vi "List-Swap Select and Un-Select.vi"(8 "error in (no error)":errorcluster, 11 "List in":refnum<vi>) -> (0 "error out":errorcluster, 3 "List Out":refnum<vi>)   [LabVIEW 2024]
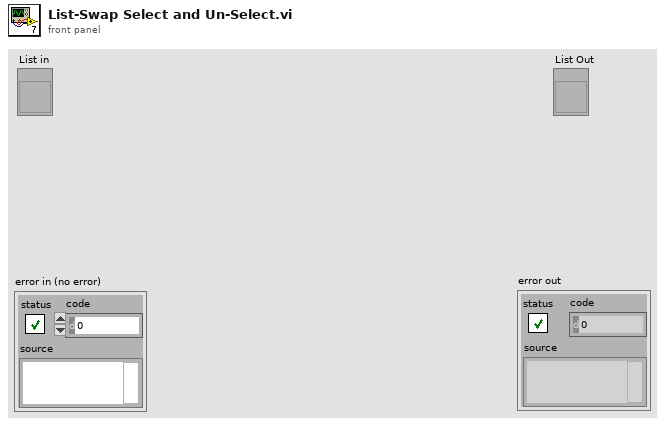
[diagram p1: front panel]
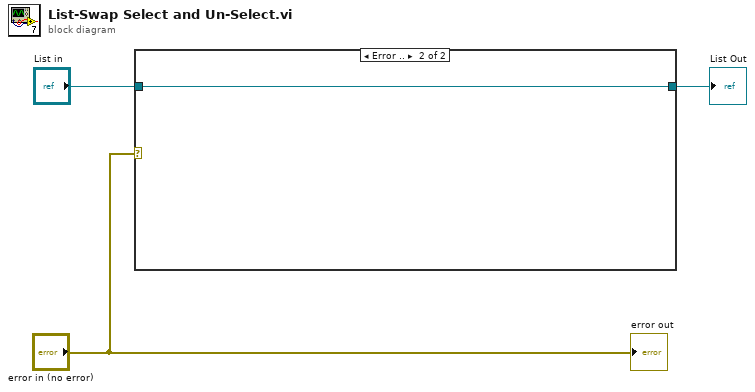
[diagram p0: block diagram]
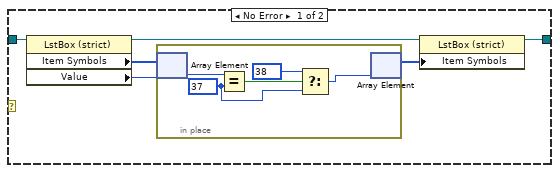
[diagram p2: hidden frame]
diagram:
  n1 = case shown="Error .." "error in (no error)" {
    tunnel: "List in" -> [w5 w15]
    tunnel: [w4 w15] -> w2
    frame No Error {
      n2 = property class="LstBox (strict)"(reference=w5) -> (reference out=w7:refnum<vi>, "Item Symbols"=w9:i32[], "Value"=w8:i32)  [unwired: 1 in, 1 out]
      n3 = in-place {
        w12 = 37
        n4 = in-place-array #1(w9, w8) -> (w14:i32)
        n5 = Equal?(x=w14, y=w12) -> (x = y?=w13:bool)
        n6 = Select(t=38, s=w13, f=w12) -> (s? t:f=w10:i32)
        n7 = in-place-array #1(w10) -> (w6:i32[])  [unwired: 1 out]
      }
      n8 = property class="LstBox (strict)"(reference=w7, "Item Symbols"=w6) -> (reference out=w4:refnum<vi>)  [unwired: 1 in, 1 out]
    }
    frame Error {
    }
  }
  "List Out" <- w2
  "error out" <- "error in (no error)"
